vi "Set Up Dialog - Hand Dynamometer.vi"() -> ()   [LabVIEW 2012]
panel:
  in  "Done":bool
  # "iWorx - Hand Dynamometer - Set Up"
  # "Set Up Instructions"
  # "1. Connect the IX-MYDAQ Sensor Adaptor into the NI myDAQ. \n\n2. Connect the GPSN-100 Gas Pressure sensor to the IX-MYDAQ.\n\n3. Connect the NI myDAQ to your PC using a USB cable.\n \n4. Connect the FT-220 to the GPSN-100 using the A-BT-220 tubing provided."
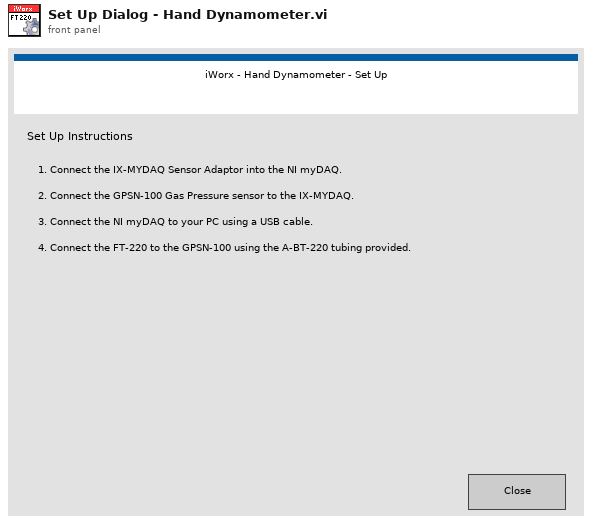
[diagram p1: front panel]
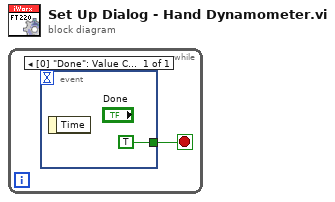
[diagram p0: block diagram]
diagram:
  n1 = while {
    stop <- w1 stop-if-true
    n2 = event shown="[0] \"Done\": Value Change;  Panel Close" {
      selector: _ -> [_]
      dyn-events: _ -> [_]
      timeout: _ -> [_]
      tunnel: [TRUE] -> w1
      event "Done": Value Change; Panel Close {
        n3 = event-data() -> ()  [unwired: 1 in, 1 out]
      }
    }
  }
